vi "set app font.vi"(10 "parameters":variant[](array[variant]), 11 "vis":refnum<vi>[](array[refnum])) -> (0 "error report":errorcluster[](array[cluster]))   [LabVIEW 2013]
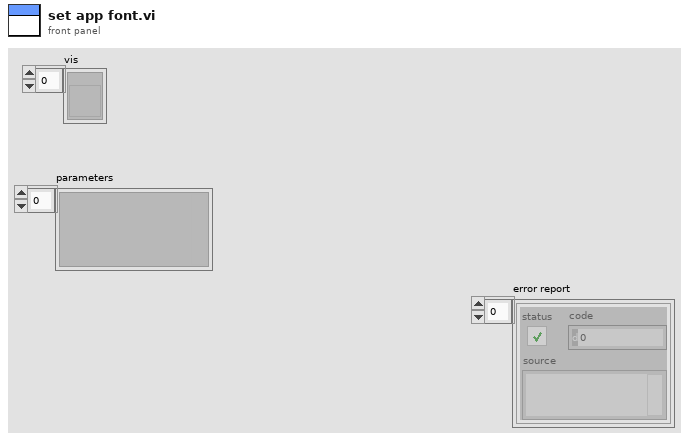
[diagram p1: front panel]
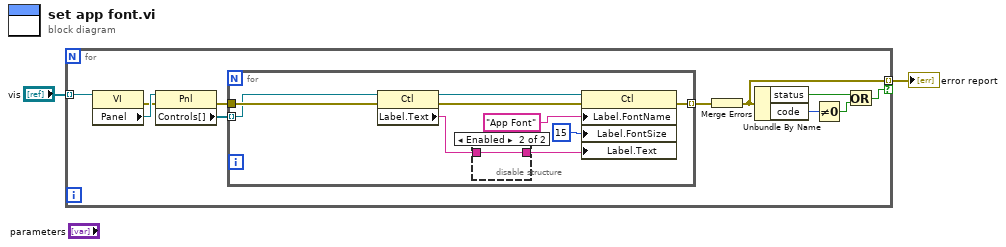
[diagram p0: block diagram]
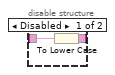
[diagram p2: hidden frame]
diagram:
  n1 = for {
    tunnel: "vis" -> [w13] mode=indexing
    tunnel: [w3] -> w1 mode=indexing if=w9
    n2 = property class="VI"(reference=w13) -> (error out=w4:errorcluster, "Panel"=w8:refnum<vi>)  [unwired: 1 in, 1 out]
    n3 = property class="Pnl"(reference=w8, error in=w4) -> (error out=w6:errorcluster, "Controls[]"=w7:refnum<vi>[])  [unwired: 1 out]
    n4 = for {
      tunnel: w7 -> [w17] mode=indexing
      tunnel: [w20] -> w5 mode=indexing
      tunnel: w6 -> [w19]
      n5 = property class="Ctl"(reference=w17, error in=w19) -> (reference out=w16:refnum<vi>, error out=w18:errorcluster, "Label.Text"=w15:string)
      n6 = disable-structure shown="Enabled" {
        disable-tunnel: w15 -> [w24 w25]
        disable-tunnel: [w23 w25] -> w14
        frame Disabled {
          n7 = To Lower Case(string=w24) -> (all lower case string=w23:string)
        }
        frame Enabled {
        }
      }
      n8 = property class="Ctl"(reference=w16, error in=w18, "Label.FontName"="App Font" ("Label.Font:Name"), "Label.FontSize"=u32 15 ("Label.Font:Size"), "Label.Text"=w14) -> (error out=w20:errorcluster)  [unwired: 1 out]
    }
    n9 = Merge Errors(w5) -> (w3:errorcluster)
    n10 = Unbundle By Name(w3) -> ("status"=w12:bool, "code"=w11:i32)
    n11 = Not Equal To 0?(x=w11) -> (x != 0?=w10:bool)
    n12 = Or(x=w12, y=w10) -> (x .or. y?=w9:bool)
  }
  "error report" <- w1
